vi "Get Maximum Time.vi"(11 "Inputs":T1[](array[typedef])) -> (3 "Max Time":dbl)   [LabVIEW 2020]
uses:
  Component.ctl
  <vilib>/gmath/NI_Gmath.lvlib
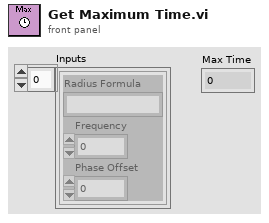
[diagram p1: front panel]
types:
  T1 = typedef "Component.ctl" = cluster{"Radius Formula":string, "Frequency":dbl, "Phase Offset":dbl}
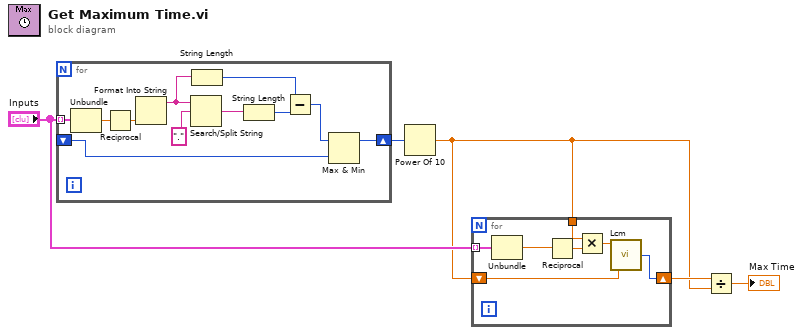
[diagram p0: block diagram]
diagram:
  n1 = for {
    tunnel: "Inputs" -> [w16] mode=indexing
    shift-right: [w9] -> w2
    shift-left: _ -> [w8]
    n2 = Unbundle(w16) -> ("Frequency"=w7:dbl)  [unwired: 2 out]
    n3 = Reciprocal(x=w7) -> (1/x=w6:dbl)
    n4 = Format Into String(w6) -> (resulting string=w13:string)  [unwired: 3 in, 1 out]
    n5 = Search/Split String(string=w13, search string/char (-)=".") -> (match + rest of string=w14:string)  [unwired: 1 in, 2 out]
    n6 = String Length(string=w13) -> (length=w11:i32)
    n7 = String Length(string=w14) -> (length=w12:i32)
    n8 = Subtract(x=w11, y=w12) -> (x-y=w10:i32)
    n9 = Max & Min(x=w10, y=w8) -> (max(x,y)=w9:i32)  [unwired: 1 out]
  }
  n10 = Power Of 10(x=w2) -> (10^x=w1:dbl)
  n11 = for {
    shift-right: [w23] -> w4
    shift-left: w1 -> [w21]
    tunnel: "Inputs" -> [w22] mode=indexing
    tunnel: w1 -> [w19]
    n12 = Unbundle(w22) -> ("Frequency"=w20:dbl)  [unwired: 2 out]
    n13 = Reciprocal(x=w20) -> (1/x=w18:dbl)
    n14 = Multiply(x=w19, y=w18) -> (x*y=w17:dbl)
    n15 = call <vilib>:"Lcm.vi"("y"=w21, "x"=w17) -> ("lcm(x,y)"=w23:i64)
  }
  n16 = Divide(x=w4, y=w1) -> (x/y=→"Max Time":dbl)
